vi "Create_New_Build.vi"(6 "buildSpecName":string, 7 "Programmatic? (false)":bool, 8 "error in (no error)":errorcluster, 9 "buildObject":T1, 10 "Destination Path":path, 11 "AB_PackedLibrary in":refnum<class "AB_PackedLibrary.lvclass">) -> (0 "error out":errorcluster, 3 "AB_PackedLibrary out":refnum<class "AB_PackedLibrary.lvclass">)   [LabVIEW 2020, in "AB_PackedLibrary.lvclass"]
uses:
  <vilib>/AppBuilder/AB_Classes/PackedLib/AB_PackedLibrary.lvclass
  e:/builds/penguin/labview/branches/2020/dev/dist/vi.lib/AppBuilder/AB_Classes/TargetFile/AB_Targetfile.lvclass
  e:/builds/penguin/labview/branches/2020/dev/dist/vi.lib/AppBuilder/AB_Classes/Build/AB_Build.lvclass
  <resource>/Framework/Providers/API/ItemRef.ctl
  <vilib>/AppBuilder/AB_Classes/PackedLib/AB_PackedLibrary.lvclass/AB_PackedLibrary.ctl
  <resource>/Framework/Providers/Common/provcom_StringGlobals.vi
  <vilib>/AppBuilder/AB_Classes/TargetFile/AB_Targetfile.lvclass
  <vilib>/AppBuilder/AB_Classes/Build/AB_Build.lvclass
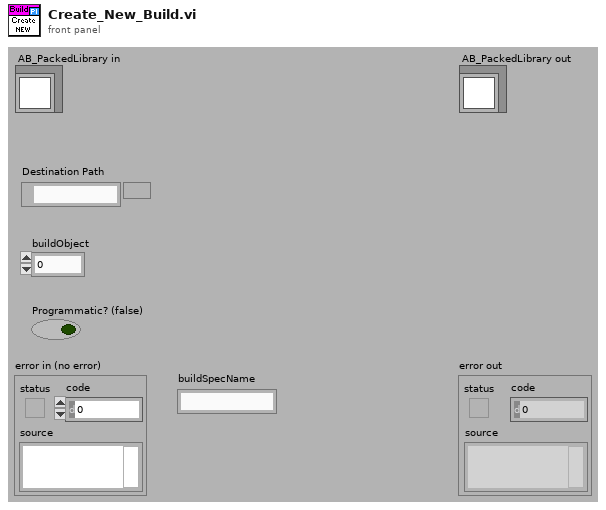
[diagram p1: front panel]
types:
  T1 = typedef "ItemRef.ctl" = u64
  T2 = typedef "AB_Targetfile.ctl" = cluster{"targetfileName":string, "targetfileGUID":string, "enableDebugging":bool, "versionInfo":cluster{"productName":string, "legalCopyright":string, "companyName":string, "internalName":string, "fileDescription":string}, "eng_consolidatedTypeInfo":string, "fastFileFormat":bool, "eng_LEIFBuildData":u32, "versionIndependent":bool}
  T3 = typedef "AB_Build.ctl" = cluster{"buildSpecName":string, "buildSpecDescription":string, "destinations":refnum<class "AB_Destination.lvclass">[], "exclusionOption":T4, "defaultLanguage":string, "supportedLanguages":string[], "excludedDirectories":path[], "buildContext":refnum<vi>, "buildObject":T1, "preview":bool, "programatic":bool, "progressBarEvents":T5, "userLog_Path":path, "preActionID":string, "preAction_Path":path, "postActionID":string, "postAction_Path":path, "eng_checkForBrokenVIs?":bool, "eng_verboseLinkerErrors?":bool, "localDest_Path":path, "targetDest_Path":path, "removeVIObject":u16, "cache":refnum<class "PreviewCache.lvclass">, "use cache":bool, "previewCache_ID":string, "buildCache_ID":string, "eng_TempLocalDest_Path":path, "eng_collectDependencies?":bool, "versionInfo":cluster{"buildVersion":cluster{"major":u16, "minor":u16, "patch":u16, "build":u16}, "autoIncrement":bool}, "eng_enableVIChecksums":bool}
  T4 = typedef "AB_Exclusion_Option.ctl" = cluster{"typedefs":bool, "polymorphicVIs":bool, "unusedLibraryItems":bool, "modifyLibraryFile":bool, "edit-timeDependencies":bool, "inlineVIs":bool, "dependent PPLs":bool, "dependent DLLs":bool}
  T5 = typedef "provcom_ProgressBar_Events.ctl" = cluster{"newJob":refnum<user-event>, "newItem":refnum<user-event>, "errorMsg":T6, "cancel":refnum<user-event>}
  T6 = typedef "mxLvBuildError.ctl" = refnum<user-event>
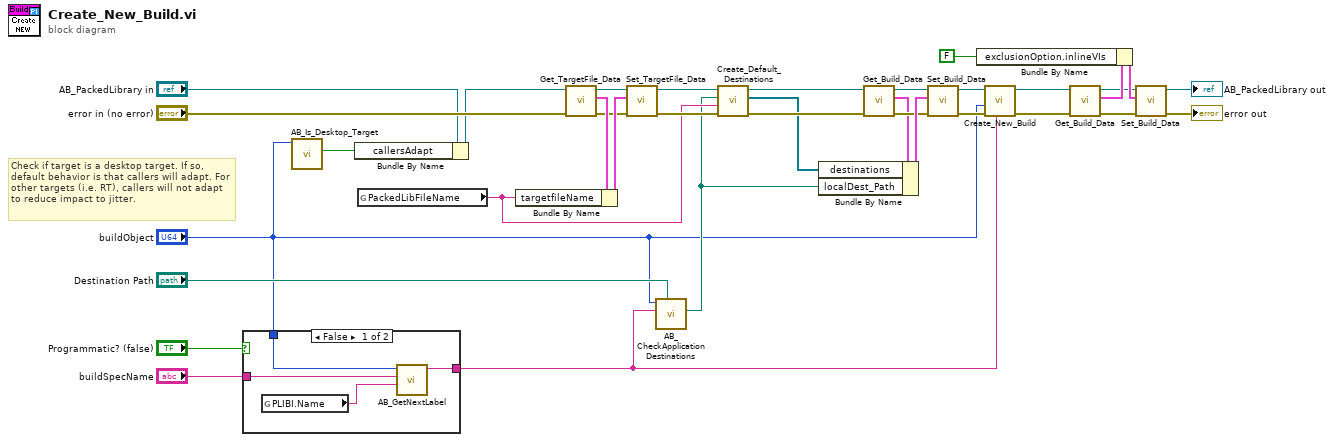
[diagram p0: block diagram]
diagram:
  # "Check if target is a desktop target. If so, default behavior is that callers will adapt. For other targets (i.e. RT), callers will not adapt to reduce impact to jitter."
  n1 = case shown="False" "Programmatic? (false)" {
    tunnel: "buildSpecName" -> [w36 w40]
    tunnel: [w39 w40] -> w12
    tunnel: "buildObject" -> [w38 _]
    frame False {
      n2 = global read "provcom_StringGlobals.vi" "PLIBI.Name"() -> (w37:string)
      n3 = call <vilib>:"AB_GetNextLabel.vi"("default name"=w37, "supplied name"=w36, "buildObject"=w38) -> ("New label"=w39:string)  [unwired: 2 in, 6 out]
    }
    frame True {
    }
  }
  n4 = call <resource>:"AB_Is_Desktop_Target.vi"("Object"="buildObject") -> ("Desktop target"=w10:bool)  [unwired: 8 in, 2 out]
  n5 = Bundle By Name(cluster="AB_PackedLibrary in", "callersAdapt"=w10) -> (w13:refnum<class "AB_PackedLibrary.lvclass">)
  n6 = global read "provcom_StringGlobals.vi" "PackedLibFileName"() -> (w16:string)
  n7 = call <vilib>:"Get_TargetFile_Data.vi"("error in (no error)"="error in (no error)", "AB_Targetfile in"=w13) -> ("error out"=w30:errorcluster, "data"=w34:T2, "AB_Targetfile out"=w32:refnum<class "AB_PackedLibrary.lvclass">)  [unwired: 7 in]
  n8 = Bundle By Name(cluster=w34, "targetfileName"=w16) -> (w33:T2)
  n9 = call <vilib>:"Set_TargetFile_Data.vi"("error in (no error)"=w30, "data"=w33, "AB_Targetfile in"=w32) -> ("error out"=w27:errorcluster, "AB_Targetfile out"=w28:refnum<class "AB_PackedLibrary.lvclass">)  [unwired: 7 in]
  n10 = call <vilib>:"AB_CheckApplicationDestinations.vi"("Destination Path"="Destination Path", "buildSpecName"=w12, "buildObject"="buildObject") -> ("Checked base path"=w15:path)  [unwired: 2 in, 6 out]
  n11 = call-dynamic "Create_Default_Destinations.vi"("error in (no error)"=w27, "Destination Name"=w16, "Destination Path"=w15, "AB_PackedLibrary in"=w28) -> ("error out"=w21:errorcluster, "default dests"=w18:refnum<class "AB_Destination.lvclass">[], "AB_PackedLibrary out"=w22:refnum<class "AB_PackedLibrary.lvclass">)  [unwired: 5 in]
  n12 = call <vilib>:"Get_Build_Data.vi"("error in (no error)"=w21, "Class in"=w22) -> ("error out"=w25:errorcluster, "data"=w23:T3, "Class out"=w24:refnum<class "AB_PackedLibrary.lvclass">)  [unwired: 7 out]
  n13 = Bundle By Name(cluster=w23, "destinations"=w18, "localDest_Path"=w15) -> (w26:T3)
  n14 = call <vilib>:"Set_Build_Data.vi"("error in (no error)"=w25, "data"=w26, "Class in"=w24) -> ("error out"=w19:errorcluster, "Class out"=w20:refnum<class "AB_PackedLibrary.lvclass">)  [unwired: 7 out]
  n15 = call-parent "Create_New_Build.vi"("buildSpecName"=w12, "error in (no error)"=w19, "buildObject"="buildObject", "AB_Targetfile in"=w20) -> ("error out"=w3:errorcluster, "AB_Targetfile out"=w5:refnum<class "AB_PackedLibrary.lvclass">)  [unwired: 2 in, 4 out]
  n16 = call <vilib>:"Get_Build_Data.vi"("error in (no error)"=w3, "Class in"=w5) -> ("error out"=w1:errorcluster, "data"=w9:T3, "Class out"=w7:refnum<class "AB_PackedLibrary.lvclass">)  [unwired: 7 out]
  n17 = Bundle By Name(cluster=w9, "exclusionOption.inlineVIs"=FALSE ("exclusionOption.modifyLibraryFile")) -> (w8:T3)
  n18 = call <vilib>:"Set_Build_Data.vi"("error in (no error)"=w1, "data"=w8, "Class in"=w7) -> ("error out"=→"error out":errorcluster, "Class out"=→"AB_PackedLibrary out":refnum<class "AB_PackedLibrary.lvclass">)  [unwired: 7 out]
